vi "Add Response_ex2.vi"() -> ()   [LabVIEW 2019]
uses:
  <vilib>/NI VeriStand/Custom Device API/Custom Device Item Ref.ctl
  Control 8.ctl
  Scripting API/Polymorphic/Add Response_Wait sec.vi
  Scripting API/Scripting API.lvlib
  <vilib>/NI VeriStand/Custom Device API/Custom Device API.lvlib
panel:
  out "Message Refnum Out":T1=18446744073709551615 format="%.0x"
  out "Response Refnum":T1=18446744073709551615 format="%.0x"
  out "Error Out":errorcluster
  in  "Message Refnum In":T1=18446744073709551615 format="%.0x"
  in  "Error In":errorcluster
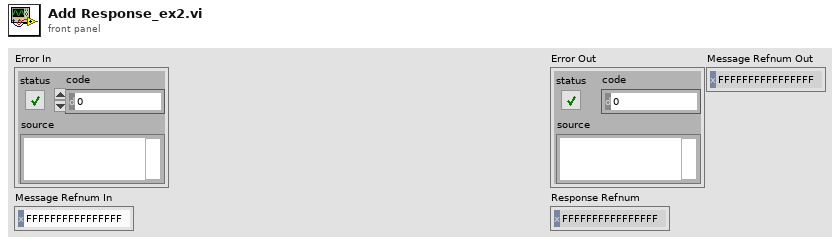
[diagram p1: front panel]
types:
  T1 = typedef "Custom Device API.lvlib/Custom Device Item Ref.ctl" = u64
  T2 = typedef "Control 8.ctl" = cluster{"Response Format":string, "Linkages":cluster{"Variable name":string, "Linked Channel refnum":T1}[], "Wait value (sec)":dbl, "Use Byte Count channel?":bool, "Channel refnum":T1}
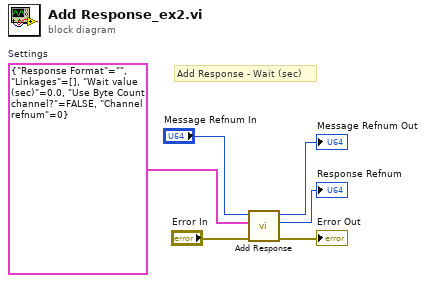
[diagram p0: block diagram]
diagram:
  w1 = T2 {"Response Format"="", "Linkages"=[], "Wait value (sec)"=0.0, "Use Byte Count channel?"=FALSE, "Channel refnum"=0}  # Settings
  # "Add Response - Wait (sec)"
  n1 = call-poly "Add Response.vi"("Error In"="Error In", "Settings"=w1, "Message Refnum In"="Message Refnum In") -> ("Error Out"=→"Error Out":errorcluster, "Response Refnum"=→"Response Refnum":T1, "Message Refnum Out"=→"Message Refnum Out":T1)  [unwired: 6 in]
